vi "Set Sif Comment.vi"(11 "comment":string) -> (2 "function return":u32, 3 "comment out":string)   [LabVIEW 2018, in "AndorSDK.lvlib"]
doc: "EXPNETTYPE unsigned int WINAPI SetSifComment(char * comment);"
uses:
  AndorSDK.lvlib
  ATMCD32D.dll
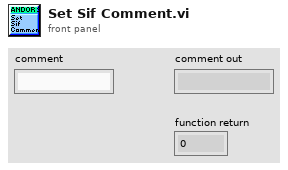
[diagram p1: front panel]
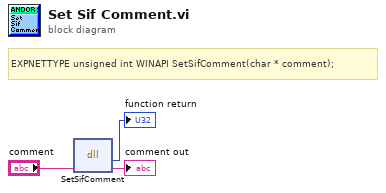
[diagram p0: block diagram]
diagram:
  # "EXPNETTYPE unsigned int WINAPI SetSifComment(char * comment);"
  n1 = dll-call lib="PTH2babs E\nPersönliches02 - Arbeit03-HiwijobsLabviewCodelibANDOR\tAndor SDK\nATMCD32D.*" fn="SetSifComment"("comment"="comment") -> (→"function return":u32, "comment"=→"comment out":string)  [unwired: 3 in, 2 out]
